vi "Set Temperature.vi"(8 "error in (no error)":errorcluster, 10 "Set Point(C)":dbl, 11 "Heating Control in":refnum<class "Heating Control.lvclass">) -> (0 "error out":errorcluster, 3 "Heating Control out":refnum<class "Heating Control.lvclass">)   [LabVIEW 2021, in "Heating Control.lvlib" / "Heating Control.lvclass"]
uses:
  Heating Control.lvclass
  C:/Program Files (x86)/National Instruments/LabVIEW 2021/vi.lib/ActorFramework/Actor/Actor.lvclass
  <vilib>/ActorFramework/Actor/Actor.lvclass/Actor.ctl
  Heating Control Interface Messages/Temp Value Changed Msg/Temp Value Changed Msg.lvclass/Temp Value Changed Msg.ctl
  <vilib>/ActorFramework/Message Enqueuer/Message Enqueuer.lvclass/Message Enqueuer.ctl
  7bc967cf-45e2-4fc3-83aa-066a887a9fd5.vi
  <vilib>/ActorFramework/Message Enqueuer/Enqueue.vi
  Heating Control Interface Messages/Temp Value Changed Msg/Temp Value Changed Msg.lvclass
  C:/Program Files (x86)/National Instruments/LabVIEW 2021/vi.lib/ActorFramework/Message/Message.lvclass
  <vilib>/ActorFramework/Message Priority Queue/Priority Enqueue.vi
  <vilib>/ActorFramework/Actor/Actor.lvclass
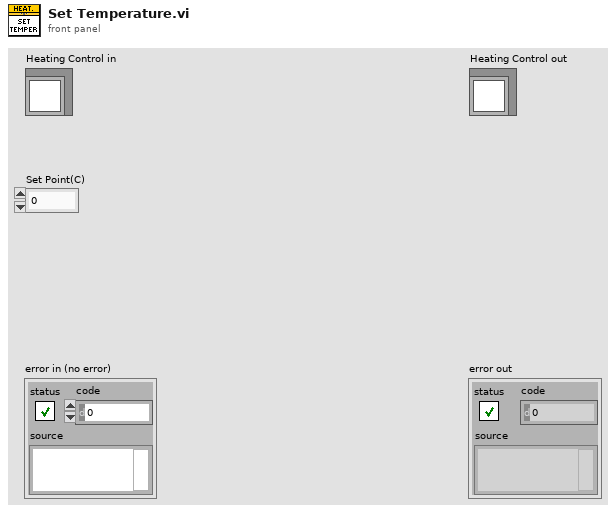
[diagram p1: front panel]
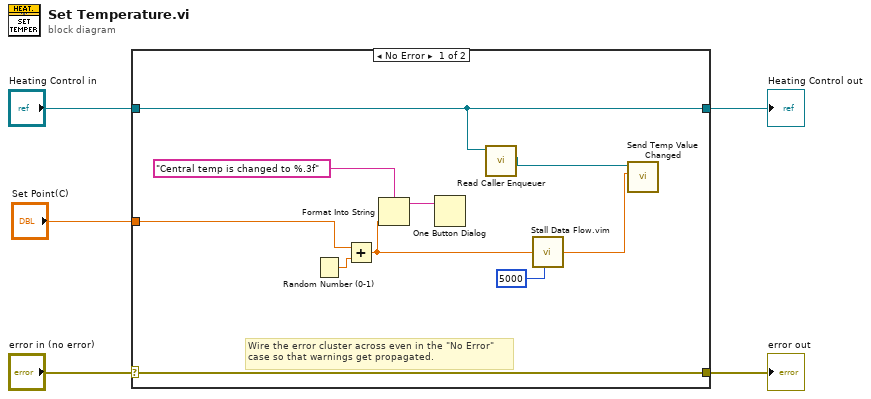
[diagram p0: block diagram]
diagram:
  n1 = case shown="No Error" "error in (no error)" {
    selector: "error in (no error)" -> [w15 w17]
    tunnel: [w15 w17] -> w4
    tunnel: [w9 w16] -> w2
    tunnel: "Heating Control in" -> [w9 w16]
    tunnel: "Set Point(C)" -> [w10 _]
    frame No Error {
      # "Wire the error cluster across even in the \"No Error\"\ncase so that warnings get propagated."
      n2 = Random Number (0-1)() -> (number: 0 to 1=w11:dbl)
      n3 = Add(x=w10, y=w11) -> (x+y=w8:dbl)
      n4 = Format Into String(format string="Central temp is changed to %.3f", w8) -> (resulting string=w13:string)  [unwired: 2 in, 1 out]
      n5 = One Button Dialog(message=w13) -> ()  [unwired: 1 in, 1 out]
      n6 = call <vilib>:"Read Caller Enqueuer.vi"("Actor"=w9) -> ("Caller Enqueuer"=w7:refnum<class "Message Enqueuer.lvclass">)  [unwired: 10 in]
      n7 = call "Stall Data Flow.vim"("value in"=w8, "milliseconds to wait"=u32 5000 ("millisecond timer value")) -> ("value out"=w6:dbl)  [unwired: 1 out]
      n8 = call "Send Temp Value Changed.vi"("Current Temp. Value"=w6, "Message Enqueuer"=w7) -> ()  [unwired: 8 in, 2 out]
    }
    frame Error {
    }
  }
  "error out" <- w4
  "Heating Control out" <- w2
